vi "oa_Get Resampled Signal Cycle by Cycle (1 Channel).vi"(0 "resampled signal":cluster{"r0":dbl, "dr":dbl, "Y":dbl[]}={"r0"=0.0, "dr"=1.0, "Y"=[]} {"r0" format="%.2p"; "dr" format="%.2p"; "Y" format="%.2f"}, 1 "reset?":bool=TRUE, 11 "error in":errorcluster) -> (4 "signal out":cluster{"r0":dbl, "dr":dbl, "Y":dbl[]}[](array[cluster]) {"r0" format="%.2p"; "dr" format="%.2p"; "Y" format="%.2f"}, 15 "error out":errorcluster)   [LabVIEW 2017, in "SoundVib_RefDataProcess.lvlib"]
uses:
  <vilib>/addons/Sound and Vibration/Order Analysis/Referece Data Processing/SoundVib_RefDataProcess.lvlib
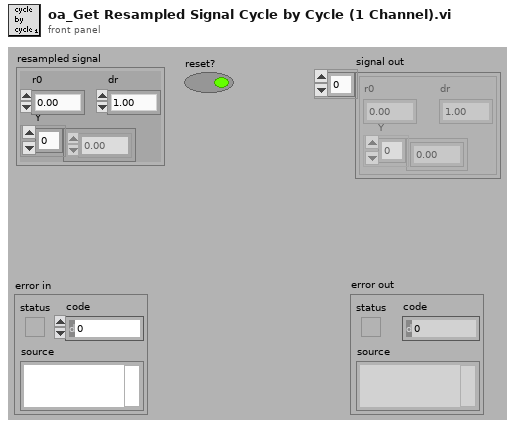
[diagram p1: front panel]
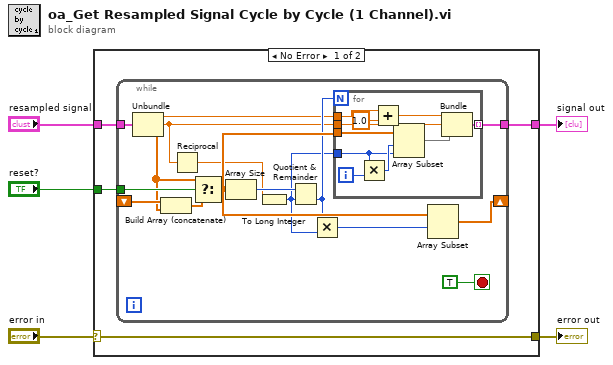
[diagram p0: block diagram]
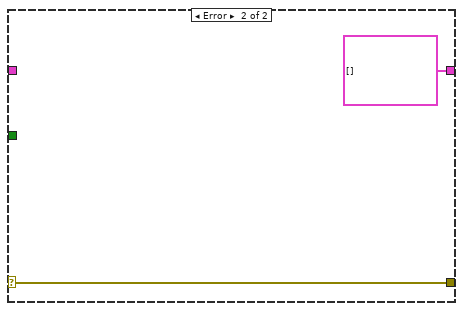
[diagram p2: hidden frame]
diagram:
  n1 = case shown="No Error" "error in" {
    selector: "error in" -> [w8 w37]
    tunnel: [w8 w37] -> w4
    tunnel: "resampled signal" -> [w9 _]
    tunnel: "reset?" -> [w7 _]
    tunnel: [w6 cluster{dbl, "dr":dbl, dbl[]}[] []] -> w1
    frame No Error {
      n2 = while {
        tunnel: w9 -> [w25]
        shift-right: [w17] -> _
        shift-left: _ -> [w21]
        tunnel: w7 -> [w22]
        tunnel: [w11] -> w6
        stop <- TRUE stop-if-true
        n3 = Unbundle(w25) -> ("r0"=w14:dbl, "dr"=w13:dbl, "Y"=w20:dbl[])
        n4 = Build Array (concatenate)(w21, w20) -> (w19:dbl[])
        n5 = Reciprocal(x=w13) -> (1/x=w12:dbl)
        n6 = Select(t=w20, s=w22, f=w19) -> (s? t:f=w16:dbl[])
        n7 = Array Size(array=w16) -> (size(s)=w24:i32)
        n8 = To Long Integer(number=w12) -> (32bit integer=w10:i32)
        n9 = Quotient & Remainder(x=w24, y=w10) -> (floor(x/y)=w15:i32)  [unwired: 1 out]
        n10 = Multiply(x=w15, y=w10) -> (x*y=w18:i32)
        n11 = for {
          N: w15 -> [_]
          tunnel: w16 -> [w35]
          tunnel: w10 -> [w28]
          tunnel: w13 -> [w31]
          tunnel: w14 -> [w29]
          tunnel: [w26] -> w11 mode=indexing
          i -> [w34]
          n12 = Multiply(x=w28, y=w34) -> (x*y=w33:i32)
          n13 = Add(x=w29, y=1.0) -> (x+y=w30:dbl)
          n14 = Array Subset(array=w35, index=w33, length=w28) -> (w32:dbl[])
          n15 = Bundle(w30, "dr"=w31, w32) -> (w26:cluster{dbl, "dr":dbl, dbl[]})  [unwired: 1 in]
        }
        n16 = Array Subset(array=w16, index=w18) -> (w17:dbl[])  [unwired: 1 in]
      }
    }
    frame Error {
    }
  }
  "error out" <- w4
  "signal out" <- w1
